vi "OAT Timebase Plot (Even Angle Signal).vi"(0 "even angle signals":cluster{"r0":dbl, "dr":dbl, "Y":dbl[]}[](array[cluster]) {"r0" format="%.2p"; "dr" format="%.2p"; "Y" format="%.2f"}, 2 "reset? (T)":bool=TRUE, 5 "speed profile":T2 {"speed [RPM]" format="%.2f"; "time [s]" format="%.2f"}, 7 "even angle position info":T3, 9 "revolutions to display [rev]":cluster{"start":dbl, "duration":dbl}={"start"=0.0, "duration"=8.0} {"duration" format="%.2f"; "start" format="%.2f"}, 11 "error in (no error)":errorcluster, 14 "trigger pulse direction":u16(ring)=1 items=["positive going", "negative going"]) -> (4 "X axis":T1, 6 "Y axis":T1, 15 "error out":errorcluster)   [LabVIEW 2017]
doc: "Draws a timebase plot on an XY graph. You can use this polymorphic VI with unfiltered or filtered data. The unfiltered data comes from the <B>even angle signals</B> input, the filtered data from the <B>magnitudes</B> and <B>phases [phase lag]</B> inputs. The timebase plot displays the amplitude of a signal as a function of time and marks the tachometer trigger point on the plot. The data type you wire to the <B>even angle signals</B> input determines the polymorphic instance to use."
uses:
  <vilib>/addons/Sound and Vibration/Order Analysis/Misc/OAT Position Info.ctl
  <vilib>/addons/Sound and Vibration/Order Analysis/Tach Process/SubVIs/speed profile.ctl
  <vilib>/addons/Sound and Vibration/Order Analysis/Backward Compatibility/SubVIs/oa_Timebase Plot Control.ctl
  <vilib>/addons/Sound and Vibration/Order Analysis/Resample Order Tracking/SoundVib_Resampling.lvlib
  <vilib>/addons/Sound and Vibration/Order Analysis/Tach Process/SoundVib_TachProcess.lvlib
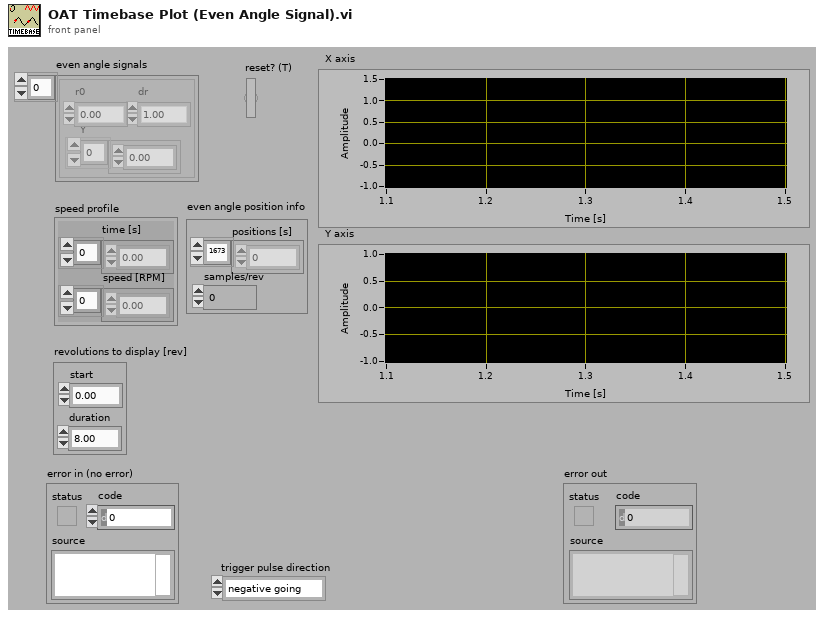
[diagram p1: front panel]
types:
  T1 = typedef "oa_Timebase Plot Control.ctl" = cluster{"X":dbl[], "Y":dbl[]}[]
  T2 = typedef "SoundVib_TachProcess.lvlib/speed profile.ctl" = cluster{"time [s]":dbl[], "speed [RPM]":dbl[]}
  T3 = typedef "OAT Position Info.ctl" = cluster{"positions [s]":dbl[], "samples/rev":dbl}
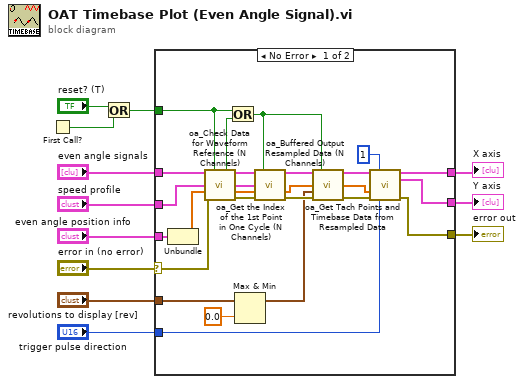
[diagram p0: block diagram]
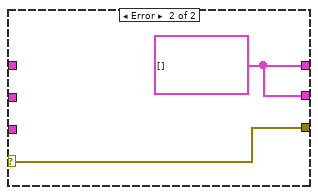
[diagram p2: hidden frame]
diagram:
  n1 = First Call?() -> (First Call?: T/F=w6:bool)
  n2 = Or(x="reset? (T)", y=w6) -> (x .or. y?=w5:bool)
  n3 = case shown="No Error" "error in (no error)" {
    selector: "error in (no error)" -> [w33 w40]
    tunnel: [w22 w40] -> w11
    tunnel: "even angle signals" -> [w34 _]
    tunnel: "speed profile" -> [w32 _]
    tunnel: "even angle position info" -> [w18 _]
    tunnel: w5 -> [w31 _]
    tunnel: "revolutions to display [rev]" -> [w28 _]
    tunnel: "trigger pulse direction" -> [w23 _]
    tunnel: [w20 w39] -> w2
    tunnel: [w19 w39] -> w1
    frame No Error {
      n4 = Unbundle(w18) -> ("positions [s]"=w17:dbl[])  [unwired: 1 out]
      n5 = call <vilib>:"oa_Check Data for Waveform Reference (N Channels).vi"("resampled signal"=w34, "reset? (True)"=w31, "speed profile"=w32, "interpolated pulse positions"=w17, "error in (no error)"=w33) -> ("reset"=w30:bool, "resampled data out"=w37:cluster{"r0":dbl, "dr":dbl, "Y":dbl[]}[], "speed profile out"=w35:T2, "interpolated pulse positions out"=w36:dbl[], "error out"=w38:errorcluster)  [unwired: 3 in, 3 out]
      n6 = Or(x=w31, y=w30) -> (x .or. y?=w26:bool)
      n7 = Max & Min(x=w28, y=0.0 ("tach duty")) -> (max(x,y)=w16:cluster{"start":dbl, "duration":dbl})  [unwired: 1 out]
      n8 = call <vilib>:"oa_Get the Index of the 1st Point in One Cycle (N Channels).vi"("resampled signal"=w37, "reset? (True)"=w26, "speed profile"=w35, "interpolated pulse positions"=w36, "error in (no error)"=w38) -> ("resampled signal out"=w29:cluster{"r0":dbl, "dr":dbl, "Y":dbl[]}[], "interpolated pulse positions out"=w14:dbl[], "error out"=w27:errorcluster)  [unwired: 8 in]
      n9 = call <vilib>:"oa_Buffered Output Resampled Data (N Channels).vi"("resampled signal in"=w29, "reset? (True)"=w26, "interpolated pulse positions"=w14, "display revolutions"=w16, "error in"=w27) -> ("resampled signal out"=w25:cluster{"r0":dbl, "dr":dbl, "Y":dbl[]}[], "interpolated pulse positions out"=w13:dbl[], "error out"=w24:errorcluster)  [unwired: 8 in]
      n10 = call <vilib>:"oa_Get Tach Points and Timebase Data from Resampled Data.vi"("resampled signal in"=w25, "tach duty"=1, "interpolated pulse positions [s]"=w13, "error in"=w24, "trigger pulse direction"=w23) -> ("X axis"=w20:cluster{dbl[], dbl[]}[], "Y axis"=w19:cluster{dbl[], dbl[]}[], "error out"=w22:errorcluster)  [unwired: 8 in]
    }
    frame Error {
      w39 = cluster{dbl[], dbl[]}[] [] ("X axis")
    }
  }
  "error out" <- w11
  "Y axis" <- w1
  "X axis" <- w2
